vi "SParameters.vi"() -> ()   [LabVIEW 2018]
doc: "PNA-X Example."
uses:
  PNA-X.lvlib
panel:
  out "XY Graph":cluster{"X Axis":dbl[], "Y Data":dbl[]}[](graph)
  in  "error in (no error)":errorcluster
  out "error out":errorcluster
  out "VISA Out":refnum<visa-resource-name>
  in  "VISA IN":refnum<visa-resource-name>
  # "1. Select Instrument Source from the \"VISA IN\" drop down.\n2. Run vi"
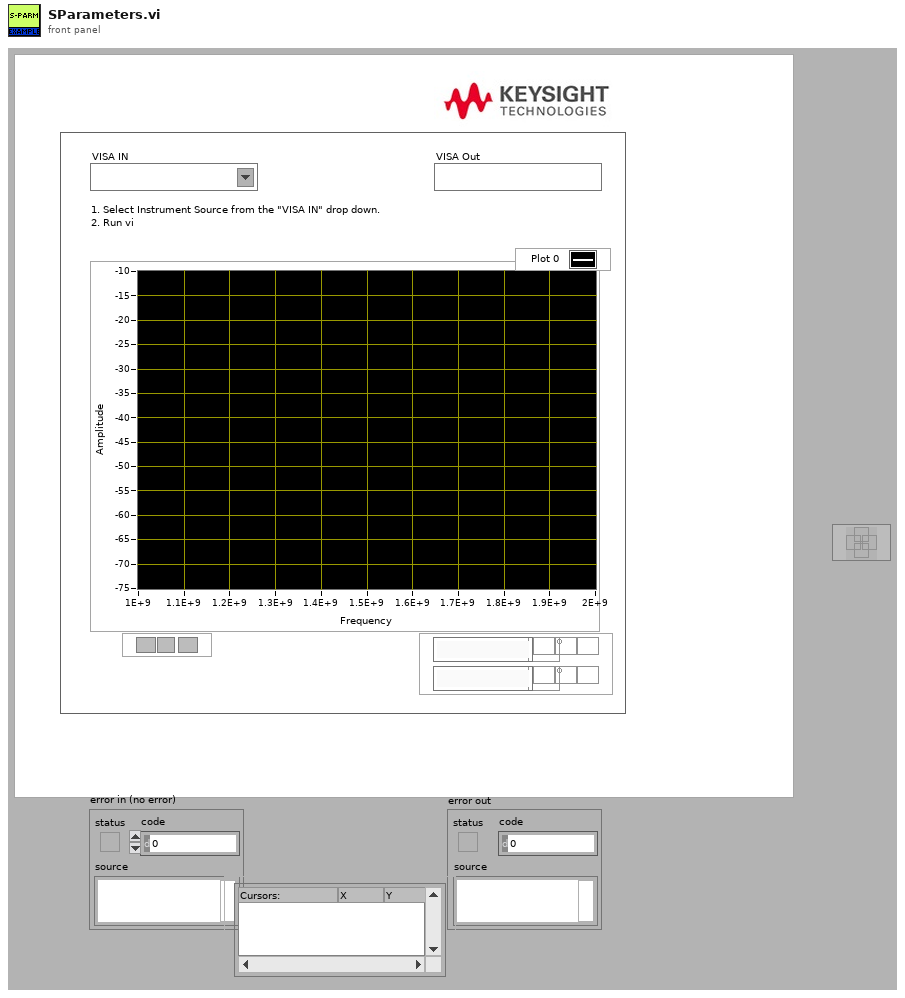
[diagram p1: front panel]
types:
  T1 = cluster{"Start Frequency":dbl, "Stop Frequency":dbl, "IF BW":dbl, "Power Level":dbl, "Format":string, "Sweep Type":string, "S11":bool, "S12":bool, "S21":bool, "S22":bool, "Autoscale?":bool, "Average?":bool, "Avg. Factor":i32, "W/Cal?":bool, "OK Button":bool}
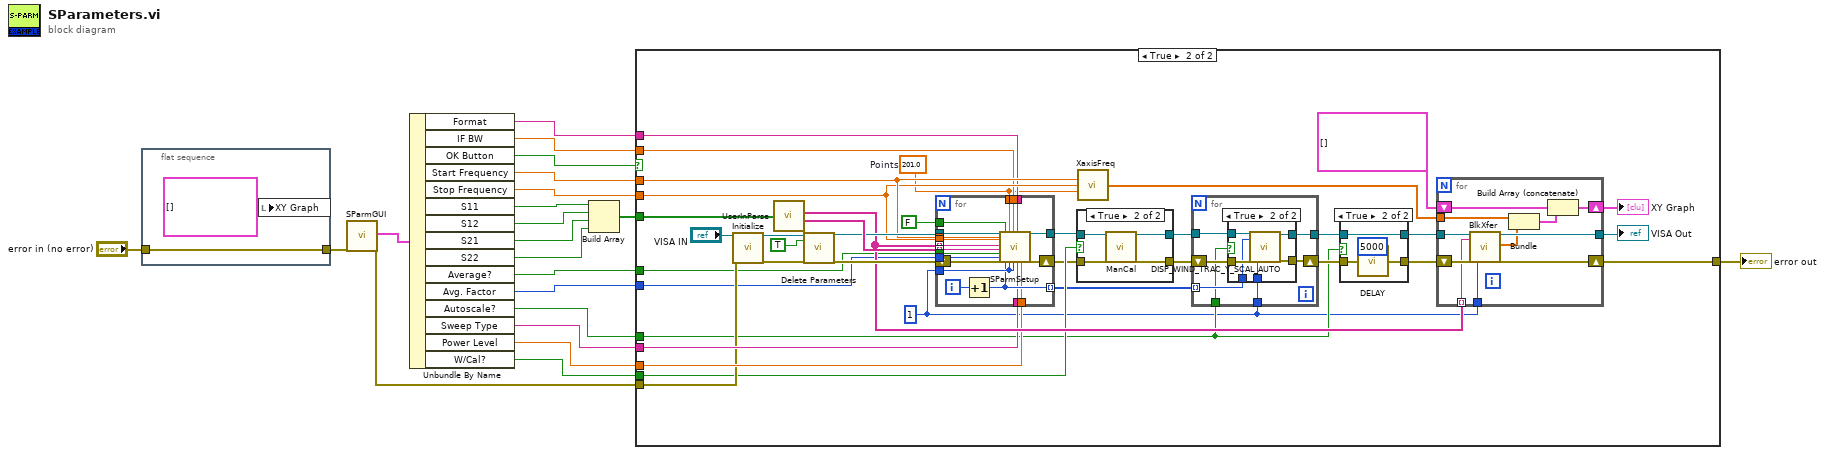
[diagram p0: block diagram]
diagram:
  n1 = flat-sequence {
    tunnel: "error in (no error)" -> [w22]
    tunnel: [w22] -> w18
    frame #0 {
      n2 = local write "XY Graph"(cluster{"X Axis":dbl[], "Y Data":dbl[]}[] [] ("XY Graph")) -> ()
    }
  }
  n3 = call "SParmGUI.vi"("error in (no error)"=w18) -> ("output cluster"=w17:T1, "error out"=w4:errorcluster)  [unwired: 17 in]
  n4 = Unbundle By Name(w17) -> ("Format"=w5:string, "IF BW"=w6:dbl, "OK Button"=w16:bool, "Start Frequency"=w15:dbl, "Stop Frequency"=w14:dbl, "S11"=w13:bool, "S12"=w12:bool, "S21"=w11:bool, "S22"=w10:bool, "Average?"=w2:bool, "Avg. Factor"=w1:i32, "Autoscale?"=w9:bool, "Sweep Type"=w8:string, "Power Level"=w7:dbl, "W/Cal?"=w3:bool)
  n5 = Build Array(w13, w12, w11, w10) -> (w20:bool[])
  n6 = case shown="True" w16 {
    tunnel: w15 -> [_ w52]
    tunnel: w14 -> [_ w51]
    tunnel: w4 -> [w24 w39]
    tunnel: w2 -> [_ w26]
    tunnel: w1 -> [_ w25]
    tunnel: [w24 w46] -> w21
    tunnel: w9 -> [_ w28]
    tunnel: w20 -> [_ w59]
    tunnel: w8 -> [_ w44]
    tunnel: w7 -> [_ w43]
    tunnel: w6 -> [_ w42]
    tunnel: w5 -> [_ w41]
    tunnel: w3 -> [_ w38]
    frame False {
    }
    frame True {
      w40 = 201.0  # Points
      w27 = 1
      n7 = call "Initialize.vi"("VISA IN"="VISA IN", "error in"=w39) -> ("VISA Out"=w57:refnum<visa-resource-name>, "error out"=w55:errorcluster)  [unwired: 15 in, 1 out]
      n8 = call "UserInParse.vi"("User Input"=w59) -> ("Filename"=w50:string[], "Measurement"=w60:string[])  [unwired: 6 in]
      n9 = call "Delete Parameters .vi"("VISA IN"=w57, "Delete All?"=TRUE, "error in"=w55) -> ("VISA Out"=w53:refnum<visa-resource-name>, "error out"=w56:errorcluster)  [unwired: 15 in]
      n10 = for {
        tunnel: w53 -> [w118]
        tunnel: [w117] -> w33
        tunnel: w52 -> [w116]
        tunnel: w51 -> [w115]
        tunnel: w50 -> [w114] mode=indexing
        tunnel: w60 -> [w113] mode=indexing
        tunnel: w26 -> [w112]
        shift-right: [w109] -> w34
        shift-left: w56 -> [w110]
        tunnel: FALSE ("Autoscale?") -> [w108]
        tunnel: w25 -> [w107]
        tunnel: w27 -> [w106]
        tunnel: [w105] -> w35 mode=indexing
        tunnel: w40 -> [w102]
        tunnel: w44 -> [w104]
        tunnel: w43 -> [w103]
        tunnel: w41 -> [w101]
        tunnel: w42 -> [w100]
        i -> [w111]
        n11 = Increment(x=w111) -> (x+1=w105:i32)
        n12 = call "SParmSetup.vi"("VISA IN"=w118, "Start Frequency"=w116, "Stop Frequency"=w115, "Filename"=w114, "Measurement"=w113, "Average?"=w112, "AVG Factor"=w107, "error in"=w110, "Autoscale?"=w108, "Trace"=w105, "Points"=w102, "Window"=w106, "IF BW"=w100, "Channel"=w106, "Format"=w101, "Sweep Type"=w104, "Power Level"=w103) -> ("VISA Out"=w117:refnum<visa-resource-name>, "error out"=w109:errorcluster)  [unwired: 9 in]
      }
      n13 = case shown="True" w38 {
        tunnel: w33 -> [w84 w88]
        tunnel: w34 -> [w83 w86]
        tunnel: [w84 w87] -> w36
        tunnel: [w83 w85] -> w37
        frame False {
        }
        frame True {
          n14 = call "ManCal.vi"("VISA IN"=w88, "error in"=w86) -> ("VISA Out"=w87:refnum<visa-resource-name>, "error out"=w85:errorcluster)  [unwired: 16 in]
        }
      }
      n15 = call "XaxisFreq.vi"("Start Frequency"=w52, "Stop Frequency"=w51, "Points"=w40) -> ("X-Axis"=w48:dbl[])  [unwired: 12 in]
      n16 = for {
        tunnel: w36 -> [w74]
        tunnel: [w71] -> w30
        tunnel: w27 -> [w70]
        tunnel: w35 -> [w69] mode=indexing
        shift-right: [w72] -> w32
        shift-left: w37 -> [w73]
        tunnel: w28 -> [w68]
        n17 = case shown="True" w68 {
          tunnel: w74 -> [w76 w82]
          tunnel: w73 -> [w75 w81]
          tunnel: [w75 w80] -> w72
          tunnel: [w76 w79] -> w71
          tunnel: w70 -> [_ w78]
          tunnel: w69 -> [_ w77]
          frame False {
          }
          frame True {
            n18 = call "DISP_WIND_TRAC_Y_SCAL_AUTO.vi"("VISA IN"=w82, "Trace"=w77, "error in"=w81, "Window"=w78) -> ("VISA Out"=w79:refnum<visa-resource-name>, "error out"=w80:errorcluster)  [unwired: 14 in]
          }
        }
      }
      n19 = case shown="True" w28 {
        tunnel: w32 -> [w62 w67]
        tunnel: [w62 w66] -> w31
        tunnel: w30 -> [w63 w64]
        tunnel: [w63 w64] -> w29
        frame False {
        }
        frame True {
          n20 = call "DELAY.vi"("milliseconds to wait"=u32 5000, "error in (no error)"=w67) -> ("error out"=w66:errorcluster)  [unwired: 13 in]
        }
      }
      n21 = for {
        tunnel: w29 -> [w99]
        tunnel: w27 -> [w97]
        tunnel: w50 -> [w96] mode=indexing
        shift-right: [w95] -> w46
        shift-left: w31 -> [w98]
        tunnel: [w94] -> w49
        tunnel: w48 -> [w92]
        shift-right: [w89] -> w47
        shift-left: cluster{"X Axis":dbl[], "Y Data":dbl[]}[] [] -> [w91]
        n22 = call "BlkXfer.vi"("VISA IN"=w99, "FileName"=w96, "error in"=w98, "Channel"=w97) -> ("VISA Out"=w94:refnum<visa-resource-name>, "Data"=w93:dbl[], "error out"=w95:errorcluster)  [unwired: 13 in]
        n23 = Bundle("X-Axis"=w92, "Data"=w93) -> (w90:cluster{"X-Axis":dbl[], "Data":dbl[]})  [unwired: 1 in]
        n24 = Build Array (concatenate)(w91, w90) -> (w89:cluster{"X-Axis":dbl[], "Data":dbl[]}[])
      }
      "VISA Out" <- w49
      "XY Graph" <- w47
    }
  }
  "error out" <- w21
